vi "Generate_HTML_Report.vi"(8 "error in (no error)":errorcluster, 11 "Working_Dir":path) -> (0 "error IO":errorcluster, 2 "HTML_Path":path, 3 "XML_Path":path)   [LabVIEW 2018, in "TestStand_Control.lvlib"]
uses:
  TestStand_Control/TestStand_Control.lvlib
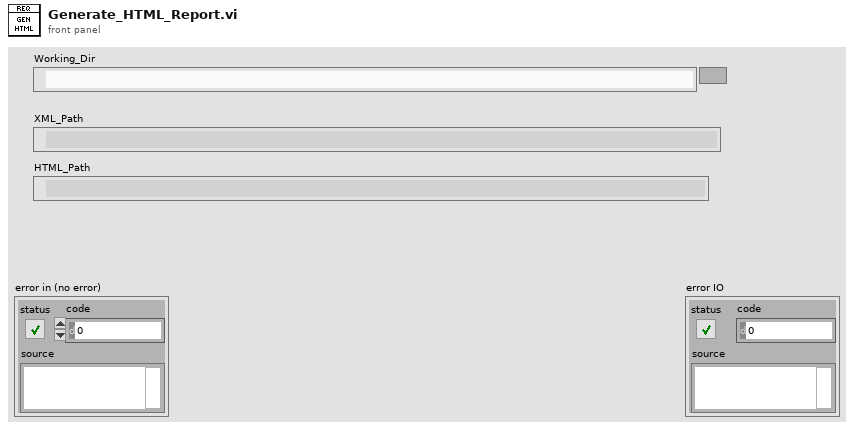
[diagram p1: front panel]
types:
  T1 = enum16{"open", "replace", "create", "open or create", "replace or create", "replace or create with confirmation"}
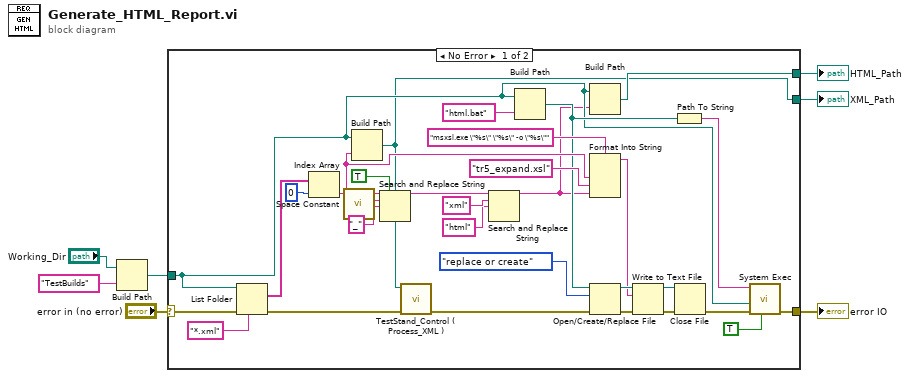
[diagram p0: block diagram]
diagram:
  n1 = Build Path(base path="Working_Dir", name or relative path="TestBuilds") -> (appended path=w2:path)
  n2 = case shown="No Error" "error in (no error)" {
    selector: "error in (no error)" -> [w30 w39]
    tunnel: [w38 _] -> w7
    tunnel: [w37 w39] -> w4
    tunnel: [w8 _] -> w5
    tunnel: w2 -> [w12 _]
    frame No Error {
      n3 = List Folder(path=w12, pattern="*.xml", error in=w30) -> (filenames=w31:string[], error out=w10:errorcluster)  [unwired: 1 in, 2 out]
      n4 = Index Array(array=w31, index=0) -> (element=w23:string)
      n5 = call <vilib>:"Space Constant.vi"() -> ("String"=w27:string)
      n6 = Build Path(base path=w12, name or relative path=w23) -> (appended path=w8:path)
      n7 = Search and Replace String(replace all?=TRUE ("replace all? (F)"), input string=w23, search string=w27, replace string="_" ("replace string (\"\")")) -> (result string=w28:string)  [unwired: 4 in, 3 out]
      n8 = call "TestStand_Control ( Process_XML ).vi"("error in"=w10, "file path (use dialog)"=w8) -> ("error out"=w9:errorcluster)  [unwired: 9 in]
      n9 = Search and Replace String(input string=w28, search string="xml", replace string="html" ("regular expression")) -> (result string=w11:string)  [unwired: 5 in, 3 out]
      n10 = Build Path(base path=w12, name or relative path="html.bat") -> (appended path=w14:path)
      n11 = Build Path(base path=w12, name or relative path=w11) -> (appended path=w38:path)
      n12 = Format Into String(format string="msxsl.exe \"%s\" \"%s\" -o \"%s\"" ("command line"), w23, "tr5_expand.xsl" ("name or relative path"), w11) -> (resulting string=w17:string)  [unwired: 2 in, 1 out]
      n13 = Open/Create/Replace File(file path (use dialog)=w14, error in=w9, operation (0:open)=T1."replace or create") -> (refnum out=w20:refnum<file>, error out=w21:errorcluster)  [unwired: 3 in, 1 out]
      n14 = Write to Text File(file (use dialog)=w20, text=w17, error in=w21) -> (refnum out=w15:refnum<file>, error out=w22:errorcluster)  [unwired: 1 in, 1 out]
      n15 = Path To String(path=w14) -> (string=w13:string)
      n16 = Close File(refnum=w15, error in=w22) -> (error out=w16:errorcluster)  [unwired: 1 out]
      n17 = call <vilib>:"System Exec.vi"("run minimized? (F)"=TRUE, "error in (no error)"=w16, "working directory"=w12, "command line"=w13) -> ("error out"=w37:errorcluster)  [unwired: 4 in, 3 out]
    }
    frame Error {
    }
  }
  "HTML_Path" <- w7
  "XML_Path" <- w5
  "error IO" <- w4
